vi "SP Enable - Disable CH Control.vi"(7 "CH Control":T1={"Trace Orientation"=enum."Overlay", "Frequency"={"Change Frequency"=FALSE, "Start"=500.0, "Stop"=1500.0, "Units"=enum."MHz"}, "Markers"=[], "Traces"=[]} {"Traces"."Reference" format="%#.2g"; "Traces"."Display Data" items=["Data", "Memory", "Data/Memory"]; "Traces"."Format" items=["Log Mag", "Phase", "Expanded Phase", "Delay", "Smith", "Polar", "Lin Mag", "SWR", "Loss", "Real", "Imaginary"]; "Traces"."Scale" min=0.001 step=1.0 format="%#.2g"; "Traces"."Position" min=0.0 max=10.0; "Frequency"."Stop" format="%.3g"; "Frequency"."Start" format="%.3g"}, 8 "error in (no error)":errorcluster, 9 "SNA? (F)":bool, 11 "CH Control Refs":refnum<vi>[](array[refnum])) -> (0 "error out":errorcluster)   [LabVIEW 2011]
uses:
  TypeDefs/SP Display Plot Controls Cluster.ctl
  TypeDefs/SP Frequency Units.ctl
  TypeDefs/SP Marker Cluster.ctl
  TypeDefs/SP Marker Type.ctl
  TypeDefs/SP Display Trace Controls.ctl
  TypeDefs/SP Display Format.ctl
  TypeDefs/SP Display Data.ctl
panel:
  # "Div"
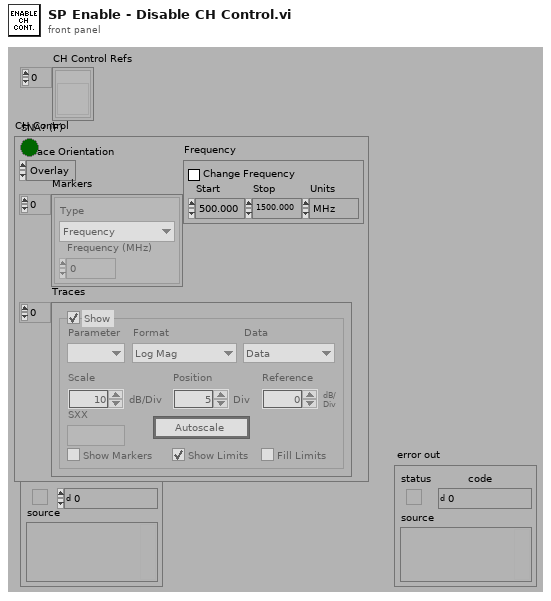
[diagram p1: front panel]
types:
  T1 = typedef "SP Display Plot Controls Cluster.ctl" = cluster{"Trace Orientation":enum32{"Overlay", "Split"}, "Frequency":cluster{"Change Frequency":bool, "Start":dbl, "Stop":dbl, "Units":T2}, "Markers":T3[], "Traces":T5[]}
  T2 = typedef "SP Frequency Units.ctl" = enum16{"Hz", "kHz", "MHz", "GHz", "Points"}
  T3 = typedef "SP Marker Cluster.ctl" = cluster{"Type":T4, "Frequency (MHz)":dbl}
  T4 = typedef "SP Marker Type.ctl" = enum16{"Frequency", "Trace Maximum", "Trace Minimum", "Limit Maximum", "Limit Minimum"}
  T5 = typedef "SP Display Trace Controls.ctl" = cluster{"Trace On":bool, "Measure":i32, "Format":T6, "Autoscale":bool, "Reference":dbl, "\nRefUnit":string, "Position":dbl, "Scale":dbl, "ScaleUnit":string, "LimitOn":bool, "LimitFill":bool, "Display Data":T7, "Show Markers":bool, "SXX":string}
  T6 = typedef "SP Display Format.ctl" = i32
  T7 = typedef "SP Display Data.ctl" = u16
  T8 = enum8{"Enabled", "Disabled", "Disabled and Grayed Out"}
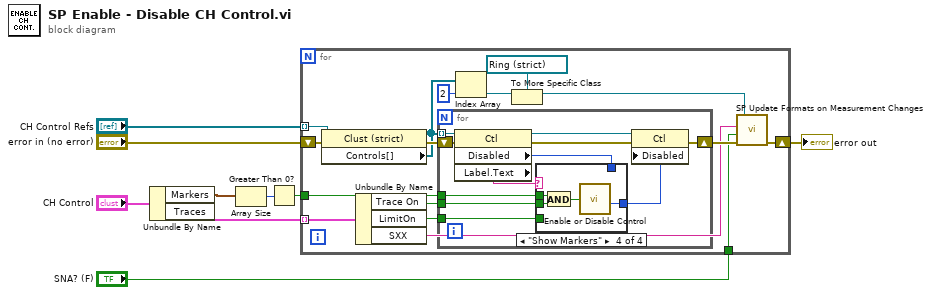
[diagram p0: block diagram]
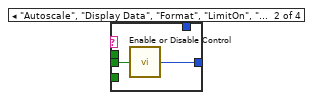
[diagram p3: hidden frame]
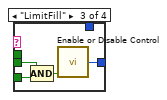
[diagram p4: hidden frame]
diagram:
  n1 = Unbundle By Name("CH Control") -> ("Markers"=w5:T3[], "Traces"=w2:T5[])
  n2 = Array Size(array=w5) -> (size(s)=w4:i32)
  n3 = Greater Than 0?(x=w4) -> (x > 0?=w3:bool)
  n4 = for {
    shift-right: [w17] -> w9
    shift-left: "error in (no error)" -> [w22]
    tunnel: "CH Control Refs" -> [w21] mode=indexing
    tunnel: w3 -> [w20]
    tunnel: w2 -> [w19] mode=indexing
    tunnel: "SNA? (F)" -> [w10]
    n5 = property class="Clust (strict)"(reference=w21, error in=w22) -> (error out=w25:errorcluster, "Controls[]"=w13:refnum<vi>[])  [unwired: 1 out]
    n6 = Unbundle By Name(w19) -> ("Trace On"=w24:bool, "LimitOn"=w23:bool, "SXX"=w11:string)
    n7 = for {
      shift-right: [w32] -> w18
      shift-left: w25 -> [w35]
      tunnel: w13 -> [w36] mode=indexing
      tunnel: w24 -> [w34]
      tunnel: w23 -> [w33]
      tunnel: w20 -> [w26]
      n8 = property class="Ctl"(reference=w36, error in=w35) -> (reference out=w31:refnum<vi>, error out=w29:errorcluster, "Disabled"=w27:u8, "Label.Text"=w28:string)
      n9 = case shown="\"Show Markers\"" w28 {
        tunnel: w34 -> [_ w39 w43 w46]
        tunnel: w33 -> [_ _ w42 _]
        tunnel: [w37 w38 w40 w47] -> w30
        tunnel: w27 -> [w37 _ _ _]
        tunnel: w26 -> [_ _ _ w44]
        frame Default {
        }
        frame "Autoscale", "Display Data", "Format", "LimitOn", "Measure", "Position", "Reference", "Scale" {
          n10 = call "Enable or Disable Control.vi"("Enable? (T)"=w39) -> ("Enable\\Disable"=w38:T8)
        }
        frame "LimitFill" {
          n11 = Compound Arithmetic op=AND(w43, w42) -> (w41:bool)
          n12 = call "Enable or Disable Control.vi"("Enable? (T)"=w41) -> ("Enable\\Disable"=w40:T8)
        }
        frame "Show Markers" {
          n13 = And(x=w44, y=w46) -> (x .and. y?=w45:bool)
          n14 = call "Enable or Disable Control.vi"("Enable? (T)"=w45) -> ("Enable\\Disable"=w47:T8)
        }
      }
      n15 = property class="Ctl"(reference=w31, error in=w29, "Disabled"=w30) -> (error out=w32:errorcluster)  [unwired: 1 out]
    }
    n16 = Index Array(array=w13, index=2) -> (element=w15:refnum<vi>)
    n17 = To More Specific Class(target class=refnum<vi> refnum ("Format"), reference=w15) -> (specific class reference=w12:refnum<vi>)  [unwired: 1 in, 1 out]
    n18 = call "SP Update Formats on Measurement Changes.vi"("error in (no error)"=w18, "SNA? (F)"=w10, "Parameter String"=w11, "Format"=w12) -> ("error out"=w17:errorcluster)  [unwired: 3 out]
  }
  "error out" <- w9
